vi "Log State.vi"(8 "error in":errorcluster, 10 "Model Status":T3, 11 "Data":T1) -> (0 "error out":errorcluster, 3 "Data out":T1)   [LabVIEW 2015, in "Logger.lvlib"]
uses:
  Logger.lvlib
  Model/TypeDefs/Get Model Status Control.ctl
  TypeDefs/Logger Data.ctl
  TypeDefs/Logger State.ctl
  Model/Model.lvlib
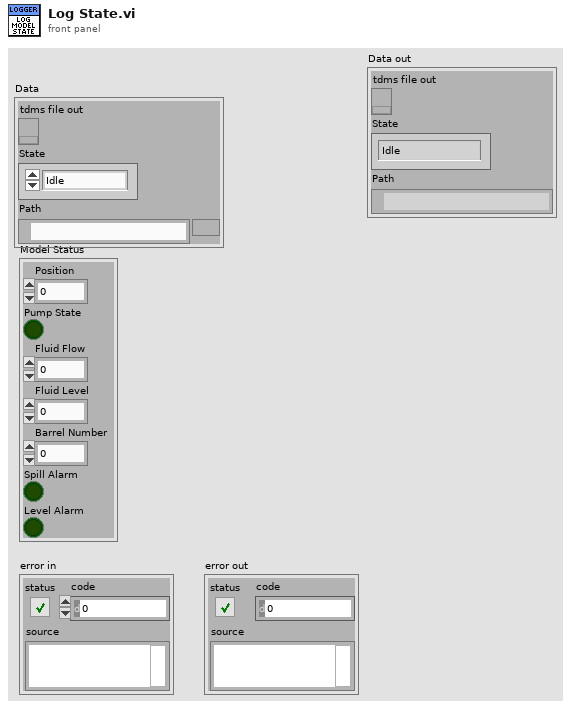
[diagram p1: front panel]
types:
  T1 = typedef "Logger.lvlib/Logger Data.ctl" = cluster{"tdms file out":refnum<k34>, "State":T2, "Path":path}
  T2 = typedef "Logger.lvlib/Logger State.ctl" = enum16{"Idle", "Working"}
  T3 = typedef "Model.lvlib/Get Model Status Control.ctl" = cluster{"Position":dbl, "Pump State":bool, "Fluid Flow":dbl, "Fluid Level":dbl, "Barrel Number":i32, "Spill Alarm":bool, "Level Alarm":bool}
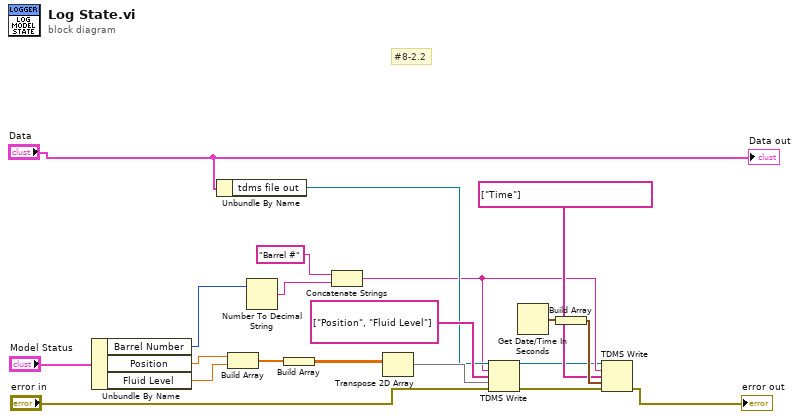
[diagram p0: block diagram]
diagram:
  # "#8-2.2"
  n1 = Unbundle By Name("Model Status") -> ("Barrel Number"=w18:i32, "Position"=w15:dbl, "Fluid Level"=w14:dbl)
  n2 = Unbundle By Name("Data") -> ("tdms file out"=w8:refnum<k34>)
  n3 = Build Array(w15, w14) -> (w13:dbl[])
  n4 = Number To Decimal String(number=w18) -> (decimal integer string=w17:string)  [unwired: 1 in]
  n5 = Build Array(w13) -> (w12:dbl[][])
  n6 = Concatenate Strings("Barrel #" ("string"), w17) -> (w4:string)
  n7 = Transpose 2D Array(2D array=w12) -> (transposed array=w10:dbl[][])
  n8 = TDMS Write(0:w8, 5:w4, 7:string[] ["Position", "Fluid Level"], 9:w10, 11:"error in") -> (4:w1:refnum<k34>, 15:w3:errorcluster)  [unwired: 1 in, 2 out]
  n9 = Get Date/Time In Seconds() -> (seconds since 1Jan1904=w7:timestamp)
  n10 = Build Array(w7) -> (w6:timestamp[])
  n11 = TDMS Write(0:w1, 5:w4, 7:string[] ["Time"], 9:w6, 11:w3) -> (15:→"error out":errorcluster)  [unwired: 1 in, 3 out]
  "Data out" <- "Data"
